vi "Parse Next I2C Linux.vi"(8 "error in (no error)":errorcluster, 10 "Bytes in":u8[](array[numeric]), 11 "pcap Parse and Build in":refnum<class "pcap_Parse_Build_CIF.lvclass">) -> (0 "error out":errorcluster, 1 "Payload":u8[](array[numeric]) format="%.0x", 2 "7 bit Address":u8, 3 "pcap Parse and Build out":refnum<class "pcap_Parse_Build_CIF.lvclass">, 4 "Bus":u8 format="%.0x", 5 "Read":bool, 6 "TAI Time (ns)":i64)   [LabVIEW 2021, in "pcap_Parse_Build_CIF.lvclass"]
uses:
  pcap_Parse_Build_CIF.lvclass
  pcap_Parse_Build_CIF.lvclass/pcap_Parse_Build_CIF.ctl
  Parse/Unflatten Packet Header.vi
  Parse/Unflatten I2C Linux Header.vi/241affe9-119b-4122-8cbe-bc40c9af6f32.vi
  Utilities/Add Error.vi
  Parse/Unflatten Packet Header.vi/a43927ee-7cb0-4c47-8c72-c2f3daaaf6fd.vi
  Data Accessors/Read Endian Match.vi
  Parse/Unflatten I2C Linux Header.vi/241affe9-119b-4122-8cbe-bc40c9af6f32.vi/c28b0ead-42ad-4072-80a2-aca7f2bd7ce3.vi
  <vilib>/CIF Foundation/CIF Utilities/Errors/Append Error Location.vi
  Parse/Unflatten Packet Header.vi/a43927ee-7cb0-4c47-8c72-c2f3daaaf6fd.vi/c28b0ead-42ad-4072-80a2-aca7f2bd7ce3.vi
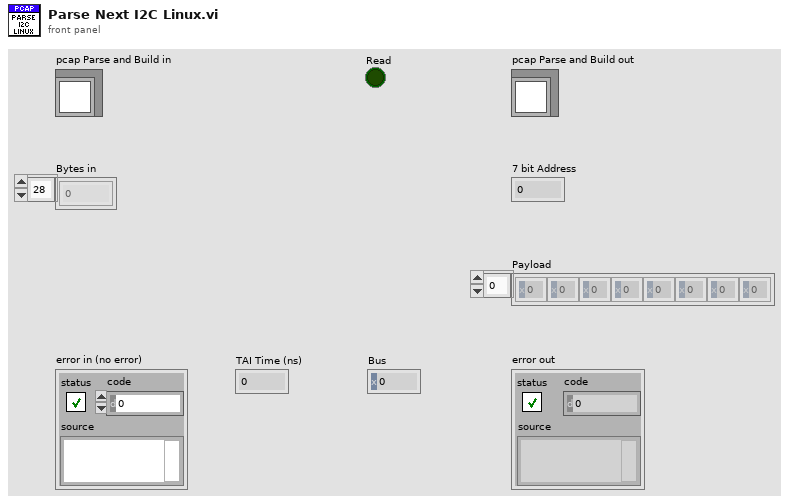
[diagram p1: front panel]
types:
  T1 = typedef "pcap_Parse_Build_CIF.lvclass/Packet Header.ctl" = cluster{"Timestamp (s)":u32, "Timestamp (ns)":u32, "Inc Length":u32, "Orig Length":u32}
  T2 = typedef "pcap_Parse_Build_CIF.lvclass/I2C Linux Header.ctl" = cluster{"Bus Number and Event Flag":u8, "Flags":u32, "HW Address":u8}
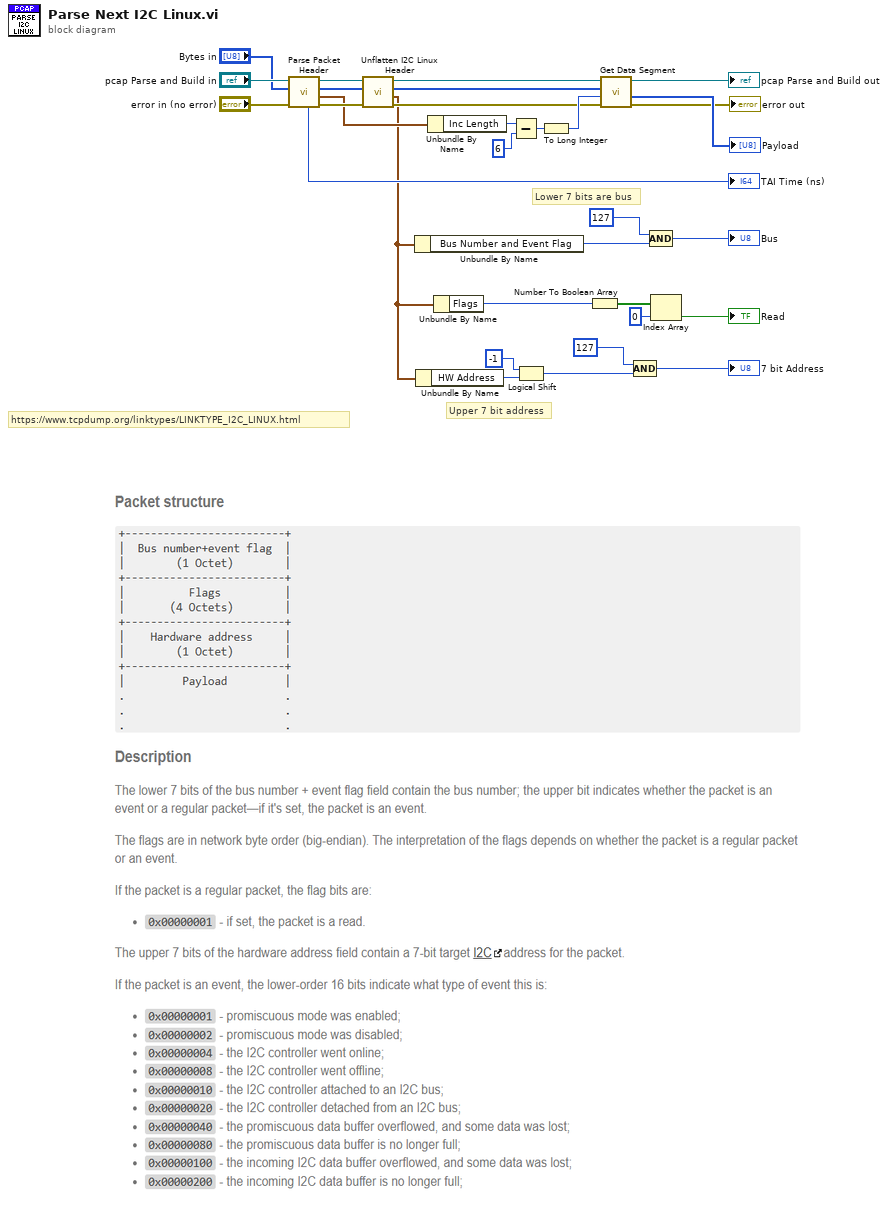
[diagram p0: block diagram]
diagram:
  # "Upper 7 bit address"
  # "https://www.tcpdump.org/linktypes/LINKTYPE_I2C_LINUX.html"
  # "Lower 7 bits are bus"
  n1 = call "Parse Packet Header.vi"("error in (no error)"="error in (no error)", "Bytes in"="Bytes in", "pcap Parse and Build in"="pcap Parse and Build in") -> ("error out"=w15:errorcluster, "Packet Header"=w13:T1, "Bytes out"=w19:u8[], "pcap Parse and Build out"=w18:refnum<class "pcap_Parse_Build_CIF.lvclass">, "TAI Time (ns)"=→"TAI Time (ns)":i64)  [unwired: 3 in, 1 out]
  n2 = call "Unflatten I2C Linux Header.vi"("error in (no error)"=w15, "Bytes in"=w19, "pcap Parse and Build in"=w18) -> ("error out"=w14:errorcluster, "I2C Lunix Header Out"=w8:T2, "Bytes out"=w16:u8[], "pcap Parse and Build out"=w17:refnum<class "pcap_Parse_Build_CIF.lvclass">)  [unwired: 5 in]
  n3 = Unbundle By Name(w8) -> ("Bus Number and Event Flag"=w9:u8)
  n4 = Unbundle By Name(w8) -> ("HW Address"=w6:u8)
  n5 = Unbundle By Name(w13) -> ("Inc Length"=w12:u32)
  n6 = Unbundle By Name(w8) -> ("Flags"=w29:u32)
  n7 = Subtract(x=w12, y=u32 6) -> (x-y=w11:u32)
  n8 = Logical Shift(y=i16 -1, x=w6) -> (x << y=w4:u8)
  n9 = To Long Integer(number=w11) -> (32bit integer=w25:i32)
  n10 = Number To Boolean Array(number=w29) -> (Boolean array=w28:bool[])
  n11 = call "Get Data Segment.vi"("error in (no error)"=w14, "Length"=w25, "Bytes in"=w16, "pcap Parse and Build in"=w17) -> ("error out"=→"error out":errorcluster, "Data Segment"=→"Payload":u8[], "pcap Parse and Build out"=→"pcap Parse and Build out":refnum<class "pcap_Parse_Build_CIF.lvclass">)  [unwired: 4 in, 1 out]
  n12 = Compound Arithmetic op=AND(u8 127 ("number"), w4) -> (→"7 bit Address":u8)
  n13 = Compound Arithmetic op=AND(u8 127 ("number"), w9) -> (→"Bus":u8)
  n14 = Index Array(array=w28, index=0) -> (element=→"Read":bool)
